vi "pf_RangeMap_to_I16.vi"(8 "error in (no error)":errorcluster, 9 "Min Range":sgl=600.0, 10 "Raw RangeMap":sgl[][](array[numeric]), 11 "Image IN":T1) -> (0 "error out":errorcluster, 3 "Image OUT":T1)   [LabVIEW 2012]
uses:
  <vilib>/vision/Image Controls.llb/IMAQ Image.ctl
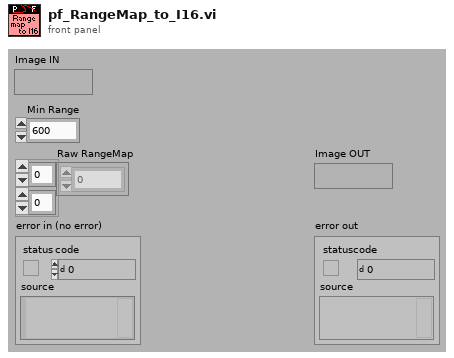
[diagram p1: front panel]
types:
  T1 = typedef "IMAQ Image.ctl" = refnum<image>
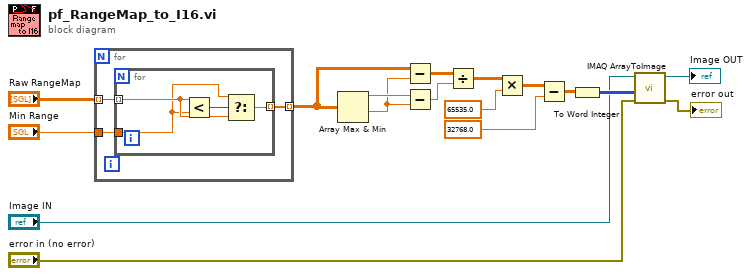
[diagram p0: block diagram]
diagram:
  n1 = for {
    tunnel: "Raw RangeMap" -> [w20] mode=indexing
    tunnel: [w19] -> w6 mode=indexing
    tunnel: "Min Range" -> [w18]
    n2 = for {
      tunnel: w20 -> [w23] mode=indexing
      tunnel: [w22] -> w19 mode=indexing
      tunnel: w18 -> [w21]
      n3 = Less?(x=w23, y=w21) -> (x < y?=w24:bool)
      n4 = Select(t=w21, s=w24, f=w23) -> (s? t:f=w22:sgl)
    }
  }
  n5 = Array Max & Min(array=w6) -> (max value=w16:sgl, min value=w15:sgl)  [unwired: 2 out]
  n6 = Subtract(x=w6, y=w15) -> (x-y=w17:sgl[][])
  n7 = Subtract(x=w16, y=w15) -> (x-y=w14:sgl)
  n8 = Divide(x=w17, y=w14) -> (x/y=w13:sgl[][])
  n9 = Multiply(x=w13, y=sgl 65535.0) -> (x*y=w12:sgl[][])
  n10 = Subtract(x=w12, y=sgl 32768.0 ("Constant")) -> (x-y=w9:sgl[][])
  n11 = To Word Integer(number=w9) -> (16bit integer=w7:i16[][])
  n12 = call "IMAQ ArrayToImage"("error in (no error)"="error in (no error)", "Image Pixels (I16)"=w7, "Image"="Image IN") -> ("error out"=→"error out":errorcluster, "Image Out"=→"Image OUT":T1)  [unwired: 3 in, 4 out]
